vi "VI Tree.vi"   [LabVIEW 2009, in "Agilent 81150.lvlib"]
doc: "This is the instrument driver for the Agilent 81150. The VI Tree displays all the user-callable VIs of the instrument driver in an organized table."
uses:
  Agilent 81150.lvlib
  Configure/Configure External Modulation Source (Amplitude).vi
  Configure/Configure Modulation (Amplitude).vi
panel:
  # "(c) 2008-2013 National Instruments.  ALL RIGHTS RESERVED."
  # "SEE DIAGRAM\nFOR VI TREE."
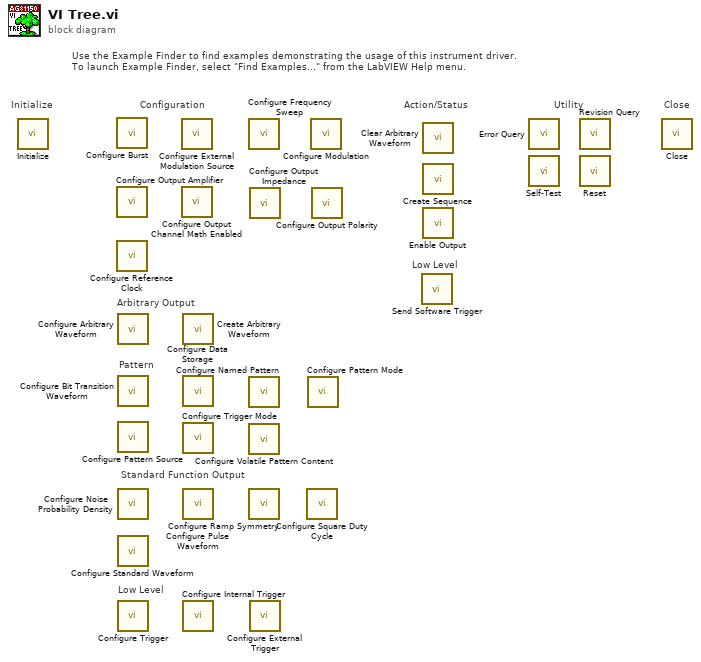
[diagram p0: block diagram]
diagram:
  # "Standard Function Output"
  # "Pattern"
  # "Arbitrary Output"
  # "Low Level"
  # "Low Level"
  # "Use the Example Finder to find examples demonstrating the usage of this instrument driver.\nTo launch Example Finder, select \"Find Examples...\" from the LabVIEW Help menu."
  # "Configuration"
  # "Utility"
  # "Action/Status"
  # "Close"
  # "Initialize"
  n1 = call "Initialize.vi"() -> ()  [unwired: 10 in, 2 out]
  n2 = call "Configure Burst.vi"() -> ()  [unwired: 10 in, 2 out]
  n3 = call "Configure Output Amplifier.vi"() -> ()  [unwired: 10 in, 2 out]
  n4 = call "Configure Reference Clock.vi"() -> ()  [unwired: 10 in, 2 out]
  n5 = call "Configure Arbitrary Waveform.vi"() -> ()  [unwired: 10 in, 2 out]
  n6 = call "Configure Bit Transition Waveform.vi"() -> ()  [unwired: 10 in, 2 out]
  n7 = call "Configure Pattern Source.vi"() -> ()  [unwired: 14 in, 2 out]
  n8 = call "Configure Noise Probability Density.vi"() -> ()  [unwired: 10 in, 2 out]
  n9 = call "Configure Standard Waveform.vi"() -> ()  [unwired: 10 in, 2 out]
  n10 = call "Configure Trigger.vi"() -> ()  [unwired: 10 in, 2 out]
  n11 = call-poly "Configure External Modulation Source.vi"() -> ()  [unwired: 10 in, 2 out]
  n12 = call "Configure Output Channel Math Enabled.vi"() -> ()  [unwired: 10 in, 2 out]
  n13 = call "Create Arbitrary Waveform.vi"() -> ()  [unwired: 10 in, 2 out]
  n14 = call "Configure Data Storage.vi"() -> ()  [unwired: 10 in, 2 out]
  n15 = call "Configure Trigger Mode.vi"() -> ()  [unwired: 10 in, 2 out]
  n16 = call "Configure Pulse Waveform.vi"() -> ()  [unwired: 10 in, 2 out]
  n17 = call "Configure Internal Trigger.vi"() -> ()  [unwired: 10 in, 2 out]
  n18 = call "Configure Frequency Sweep.vi"() -> ()  [unwired: 14 in, 2 out]
  n19 = call "Configure Named Pattern.vi"() -> ()  [unwired: 10 in, 2 out]
  n20 = call "Configure Volatile Pattern Content.vi"() -> ()  [unwired: 10 in, 2 out]
  n21 = call "Configure Ramp Symmetry.vi"() -> ()  [unwired: 10 in, 2 out]
  n22 = call "Configure Output Impedance.vi"() -> ()  [unwired: 10 in, 2 out]
  n23 = call "Configure External Trigger.vi"() -> ()  [unwired: 10 in, 2 out]
  n24 = call "Configure Square Duty Cycle.vi"() -> ()  [unwired: 10 in, 2 out]
  n25 = call "Configure Pattern Mode.vi"() -> ()  [unwired: 10 in, 2 out]
  n26 = call-poly "Configure Modulation.vi"() -> ()  [unwired: 14 in, 2 out]
  n27 = call "Configure Output Polarity.vi"() -> ()  [unwired: 10 in, 2 out]
  n28 = call "Send Software Trigger.vi"() -> ()  [unwired: 10 in, 2 out]
  n29 = call "Clear Arbitrary Waveform.vi"() -> ()  [unwired: 10 in, 2 out]
  n30 = call "Create Sequence.vi"() -> ()  [unwired: 10 in, 2 out]
  n31 = call "Enable Output.vi"() -> ()  [unwired: 10 in, 2 out]
  n32 = call "Error Query.vi"() -> ()  [unwired: 8 in, 4 out]
  n33 = call "Self-Test.vi"() -> ()  [unwired: 8 in, 4 out]
  n34 = call "Revision Query.vi"() -> ()  [unwired: 8 in, 4 out]
  n35 = call "Reset.vi"() -> ()  [unwired: 10 in, 2 out]
  n36 = call "Close.vi"() -> ()  [unwired: 11 in, 1 out]
